vi "PID-Parameter Druckregler einstellen.vi"() -> ()   [LabVIEW 2020, in "Erweiterte Konfig.lvlib"]
uses:
  Erweiterte Konfig.lvlib
  Visualisierungs Elemente/Button.ctl
  Visualisierungs Elemente/Zahlen-Eingabefeld.ctl
  Visualisierungs Elemente/Zahlen-Ausgabefeld.ctl
  cRIO/PC/Aktionen FGV Druckregler.ctl
  cRIO/PC/Kommunikation mit cRIO.lvlib
  Allgemein/allgemeine Sub-VIs.lvlib
panel:
  in  "BEENDEN":T1
  in  "Ausgang Regler -":T2 format="%#_5g"
  in  "Ausgang Regler +":T2 format="%#_5g"
  in  "Ausgang D":T2 format="%#_5g"
  in  "Ausgang I":T2 format="%#_5g"
  in  "Ausgang P":T2 format="%#_5g"
  in  "Ausgang Regler Toleranz":bool
  out "Ausgang Sollwert":T3 format="%.1f"
  out "Ausgang Istwert":T3 format="%.1f"
  out "Ausgang Regler Ausgang":T3 format="%.2f"
  out "Ausgang Analog Ausgang":T3 format="%.2f"
  out "Ausgang Integral":T3 format="%.2f"
  out "Ausgang Derivative":T3 format="%.2f"
  out "Ausgang":sgl[][](graph)
  out "FT-IR":sgl[][](graph)
  out "Pumpe":sgl[][](graph)
  out "FT-IR Sollwert":T3 format="%.2f"
  out "FT-IR Istwert":T3 format="%.2f"
  out "FT-IR Regler Ausgang":T3 format="%.2f"
  out "FT-IR Analog Ausgang":T3 format="%.2f"
  out "FT-IR Integral":T3 format="%.2f"
  out "FT-IR Derivative":T3 format="%.2f"
  out "Pumpe Derivative":T3 format="%.2f"
  out "Pumpe Integral":T3 format="%.2f"
  out "Pumpe Analog Ausgang":T3 format="%.2f"
  out "Pumpe Regler Ausgang":T3 format="%.2f"
  out "Pumpe Istwert":T3 format="%.1f"
  out "Pumpe Sollwert":T3 format="%.1f"
  in  "FT-IR Regler -":T2 format="%#_5g"
  in  "FT-IR Regler +":T2 format="%#_5g"
  in  "FT-IR D":T2 format="%#_5g"
  in  "FT-IR I":T2 format="%#_5g"
  in  "FT-IR P":T2 format="%#_5g"
  in  "FT-IR Regler Toleranz":bool
  in  "Pumpe Regler -":T2 format="%#_5g"
  in  "Pumpe Regler +":T2 format="%#_5g"
  in  "Pumpe D":T2 format="%#_5g"
  in  "Pumpe I":T2 format="%#_5g"
  in  "Pumpe P":T2 format="%#_5g"
  in  "Pumpe Regler Toleranz":bool
  # "PID Parameter Druck-Regler"
  # "Druck Kalter Block"
  # "Druck Ausgang"
  # "Gaskühler"
  # "Sollwert:"
  # "Sollwert:"
  # "Sollwert:"
  # "Verstärkung KR:"
  # "Verstärkung KR:"
  # "Verstärkung KR:"
  # "Istwert:"
  # "Istwert:"
  # "Istwert:"
  # "Nachstellzeit TN:"
  # "sec"
  # "Nachstellzeit TN:"
  # "sec"
  # "Regler OUT:"
  # "Regler OUT:"
  # "Nachstellzeit TN:"
  # "Regler OUT:"
  # "sec"
  # "Analog OUT:"
  # "Analog OUT:"
  # "Analog OUT:"
  # "Vorhaltezeit TD:"
  # "Vorhaltezeit TD:"
  # "sec"
  # "sec"
  # "Vorhaltezeit TD:"
  # "sec"
  # "I-Action:"
  # "I-Action:"
  # "I-Action:"
  # "D-Action:"
  # "D-Action:"
  # "D-Action:"
  # "mbar"
  # "mbar"
  # "Regler Toleranz +:"
  # "Regler Toleranz +:"
  # "l/min"
  # "Regler Toleranz +:"
  # "Regler Toleranz -:"
  # "mbar"
  # "Regler Toleranz -:"
  # "mbar"
  # "Regler Toleranz -:"
  # "l/min"
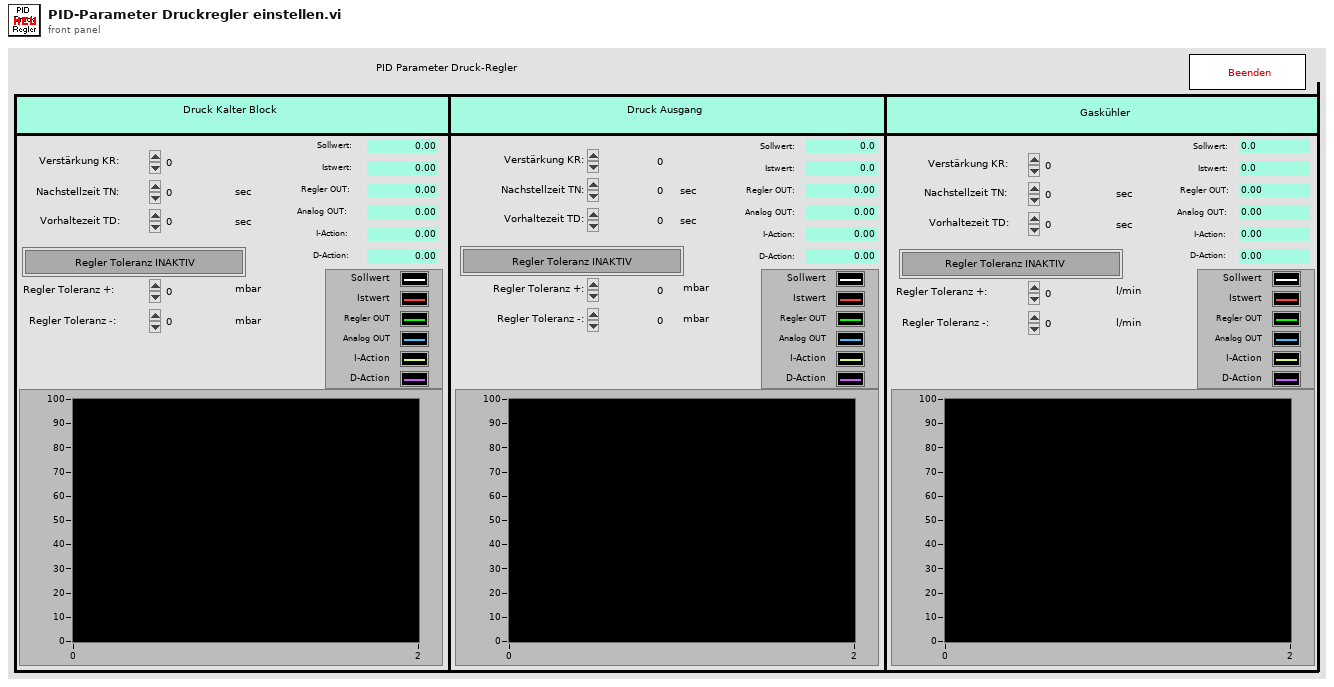
[diagram p1: front panel]
types:
  T1 = typedef "Button.ctl" = bool
  T2 = typedef "Zahlen-Eingabefeld.ctl" = sgl
  T3 = typedef "Zahlen-Ausgabefeld.ctl" = sgl
  T4 = typedef "Kommunikation mit cRIO.lvlib/Aktionen FGV Druckregler.ctl" = enum16{"lesen", "Parameter", "Istwerte"}
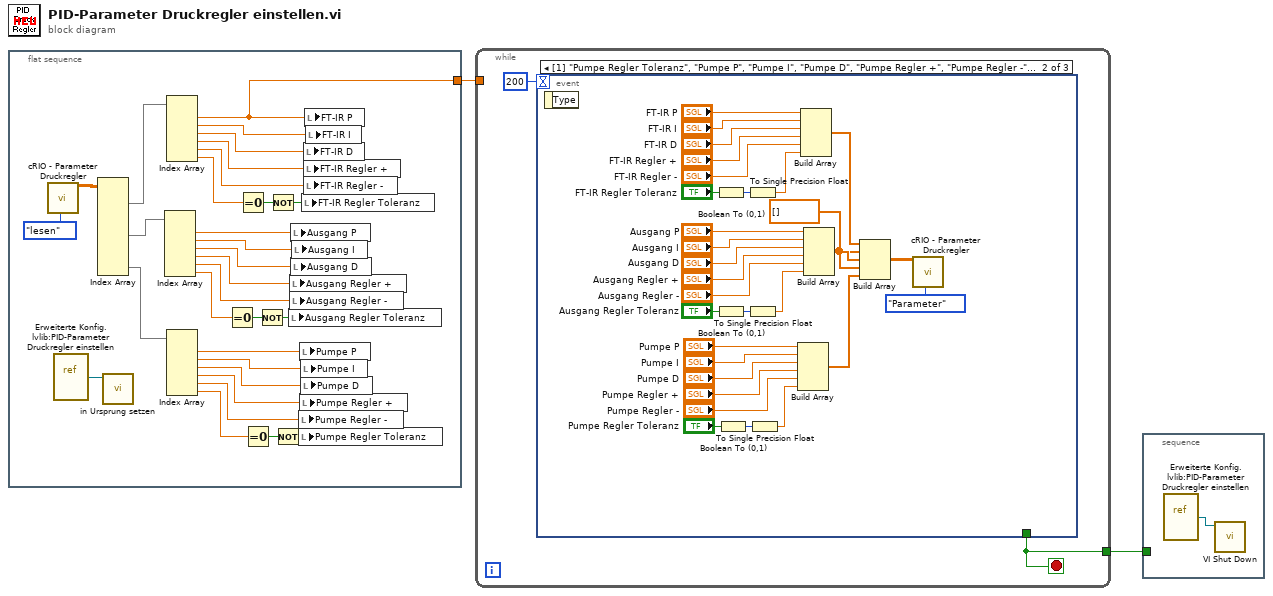
[diagram p0: block diagram]
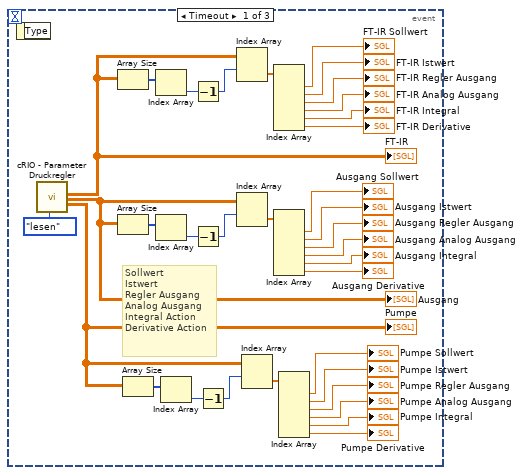
[diagram p2: hidden frame]
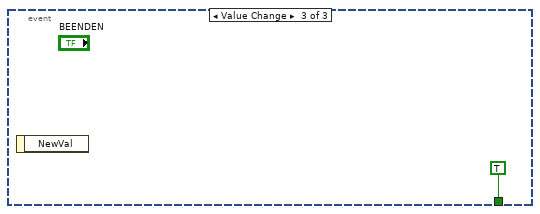
[diagram p3: hidden frame]
diagram:
  n1 = flat-sequence {
    tunnel: [w17] -> w2
    frame #0 {
      n2 = call "cRIO - Parameter Druckregler.vi"("Aktion"=Aktionen_FGV_Druckregler."lesen") -> ("Parameter Regler"=w26:sgl[][])  [unwired: 9 in, 9 out]
      n3 = vi-ref "Erweiterte Konfig.lvlib:PID-Parameter Druckregler einstellen.vi"() -> (w16:refnum<vi>)
      n4 = Index Array(array=w26) -> (element #1=w18:sgl[], element #3=w4:sgl[], element #5=w3:sgl[])  [unwired: 10 in, 2 out]
      n5 = call "in Ursprung setzen.vi"("VI Referenz"=w16) -> ()  [unwired: 11 in]
      n6 = Index Array(array=w4) -> (element #1=w23:sgl, element #2=w22:sgl, element #3=w21:sgl, element #4=w10:sgl, element #5=w9:sgl, element #6=w8:sgl)  [unwired: 6 in]
      n7 = Index Array(array=w18) -> (element #1=w17:sgl, element #2=w25:sgl, element #3=w24:sgl, element #4=w13:sgl, element #5=w12:sgl, element #6=w11:sgl)  [unwired: 6 in]
      n8 = Index Array(array=w3) -> (element #1=w28:sgl, element #2=w32:sgl, element #3=w31:sgl, element #4=w7:sgl, element #5=w6:sgl, element #6=w5:sgl)  [unwired: 6 in]
      n9 = Equal To 0?(x=w8) -> (x = 0?=w20:bool)
      n10 = Equal To 0?(x=w11) -> (x = 0?=w15:bool)
      n11 = Equal To 0?(x=w5) -> (x = 0?=w30:bool)
      n12 = Not(x=w20) -> (.not. x?=w19:bool)
      n13 = Not(x=w15) -> (.not. x?=w14:bool)
      n14 = Not(x=w30) -> (.not. x?=w29:bool)
      n15 = local write "Ausgang Regler Toleranz"(w19) -> ()
      n16 = local write "Ausgang Regler +"(w10) -> ()
      n17 = local write "Ausgang Regler -"(w9) -> ()
      n18 = local write "Ausgang P"(w23) -> ()
      n19 = local write "Ausgang D"(w21) -> ()
      n20 = local write "Ausgang I"(w22) -> ()
      n21 = local write "Pumpe Regler -"(w6) -> ()
      n22 = local write "Pumpe Regler Toleranz"(w29) -> ()
      n23 = local write "Pumpe P"(w28) -> ()
      n24 = local write "Pumpe Regler +"(w7) -> ()
      n25 = local write "Pumpe I"(w32) -> ()
      n26 = local write "Pumpe D"(w31) -> ()
      n27 = local write "FT-IR Regler Toleranz"(w14) -> ()
      n28 = local write "FT-IR D"(w24) -> ()
      n29 = local write "FT-IR Regler +"(w13) -> ()
      n30 = local write "FT-IR Regler -"(w12) -> ()
      n31 = local write "FT-IR P"(w17) -> ()
      n32 = local write "FT-IR I"(w25) -> ()
    }
  }
  n33 = while {
    tunnel: w2 -> [_]
    tunnel: [w33] -> w1
    stop <- w33 stop-if-true
    n34 = event shown="[1] \"Pumpe Regler Toleranz\", \"Pumpe P\", \"Pumpe I\", \"Pumpe D\", \"Pumpe Regler +\", \"Pumpe Regler -\", \"FT-IR Regler Toleranz\", \"FT-IR P\", \"FT-IR I\", \"FT-IR D\", \"FT-IR Regler +\", \"FT-IR Regler -\", \"Ausgang P\", \"Ausgang I\", \"Ausgang D\", \"Ausgang Regler +\", \"Ausgang Regler -\", \"Ausgang Regler Toleranz\": Wertänderung" {
      selector: _ -> [_ _ _]
      dyn-events: _ -> [_ _ _]
      timeout: 200 -> [_ _ _]
      tunnel: [_ _ TRUE ("ABBRECHEN")] -> w33
      event Timeout {
        # "Sollwert\nIstwert\nRegler Ausgang\nAnalog Ausgang\nIntegral Action\nDerivative Action"
        n35 = event-data() -> ()  [unwired: 1 in, 1 out]
        n36 = call "cRIO - Parameter Druckregler.vi"("Aktion"=Aktionen_FGV_Druckregler."lesen") -> ("Istwerte Regler FT-IR"=w35:sgl[][], "Istwerte Regler Ausgang"=w47:sgl[][], "Istwerte Regler NDIR"=w36:sgl[][])  [unwired: 9 in, 7 out]
        "FT-IR" <- w35
        "Ausgang" <- w47
        "Pumpe" <- w36
        n37 = Array Size(array=w35) -> (size(s)=w64:i32[])
        n38 = Array Size(array=w47) -> (size(s)=w63:i32[])
        n39 = Array Size(array=w36) -> (size(s)=w41:i32[])
        n40 = Index Array(array=w64) -> (element=w65:i32)  [unwired: 1 in]
        n41 = Index Array(array=w63) -> (element=w62:i32)  [unwired: 1 in]
        n42 = Index Array(array=w41) -> (element=w40:i32)  [unwired: 1 in]
        n43 = Decrement(x=w65) -> (x-1=w66:i32)
        n44 = Decrement(x=w62) -> (x-1=w61:i32)
        n45 = Decrement(x=w40) -> (x-1=w39:i32)
        n46 = Index Array(array=w35, index (row)=w66) -> (element=w67:sgl[])  [unwired: 1 in]
        n47 = Index Array(array=w47, index (row)=w61) -> (element=w60:sgl[])  [unwired: 1 in]
        n48 = Index Array(array=w36, index (row)=w39) -> (element=w38:sgl[])  [unwired: 1 in]
        n49 = Index Array(array=w67) -> (element #1=→"FT-IR Sollwert":sgl, element #2=→"FT-IR Istwert":sgl, element #3=→"FT-IR Regler Ausgang":sgl, element #4=→"FT-IR Analog Ausgang":sgl, element #5=→"FT-IR Integral":sgl, element #6=→"FT-IR Derivative":sgl)  [unwired: 6 in]
        n50 = Index Array(array=w60) -> (element #1=→"Ausgang Sollwert":sgl, element #2=→"Ausgang Istwert":sgl, element #3=→"Ausgang Regler Ausgang":sgl, element #4=→"Ausgang Analog Ausgang":sgl, element #5=→"Ausgang Integral":sgl, element #6=→"Ausgang Derivative":sgl)  [unwired: 6 in]
        n51 = Index Array(array=w38) -> (element #1=→"Pumpe Sollwert":sgl, element #2=→"Pumpe Istwert":sgl, element #3=→"Pumpe Regler Ausgang":sgl, element #4=→"Pumpe Analog Ausgang":sgl, element #5=→"Pumpe Integral":sgl, element #6=→"Pumpe Derivative":sgl)  [unwired: 6 in]
      }
      event "Pumpe Regler Toleranz", "FT-IR Regler Toleranz", "Ausgang Regler Toleranz": Value Change {
        w69 = T2[] [] ("Element")
        n52 = event-data() -> ()  [unwired: 1 in, 1 out]
        n53 = Boolean To (0,1)(Boolean="FT-IR Regler Toleranz") -> (0, 1=w98:i16)
        n54 = Boolean To (0,1)(Boolean="Ausgang Regler Toleranz") -> (0, 1=w92:i16)
        n55 = Boolean To (0,1)(Boolean="Pumpe Regler Toleranz") -> (0, 1=w84:i16)
        n56 = To Single Precision Float(number=w98) -> (single precision float=w76:sgl)
        n57 = To Single Precision Float(number=w92) -> (single precision float=w75:sgl)
        n58 = To Single Precision Float(number=w84) -> (single precision float=w70:sgl)
        n59 = Build Array("Pumpe P", "Pumpe I", "Pumpe D", "Pumpe Regler +", "Pumpe Regler -", w70) -> (w79:T2[])
        n60 = Build Array("FT-IR P", "FT-IR I", "FT-IR D", "FT-IR Regler +", "FT-IR Regler -", w76) -> (w87:T2[])
        n61 = Build Array("Ausgang P", "Ausgang I", "Ausgang D", "Ausgang Regler +", "Ausgang Regler -", w75) -> (w86:T2[])
        n62 = Build Array(w87, w69, w86, w69, w79) -> (w85:T2[][])
        n63 = call "cRIO - Parameter Druckregler.vi"("Parameter Regler"=w85, "Aktion"=Aktionen_FGV_Druckregler."Parameter") -> ()  [unwired: 8 in, 10 out]
      }
      event Value Change {
        n64 = event-data() -> ()  [unwired: 1 in, 1 out]
      }
    }
  }
  n65 = stacked-sequence {
    tunnel: w1 -> [_]
    frame #0 {
      n66 = vi-ref "Erweiterte Konfig.lvlib:PID-Parameter Druckregler einstellen.vi"() -> (w100:refnum<vi>)
      n67 = call "VI Shut Down.vi"("VI Referenz"=w100) -> ()  [unwired: 11 in]
    }
  }
